vi "Reentrant Display Caller.vi"(9 "card #":dbl, 10 "Stop Button in":bool, 11 "Display Input":T1[](array[typedef])) -> ()   [LabVIEW 2013]
uses:
  Controls/Numeric Indicator.ctl
panel:
  out "VI out":refnum<vi>
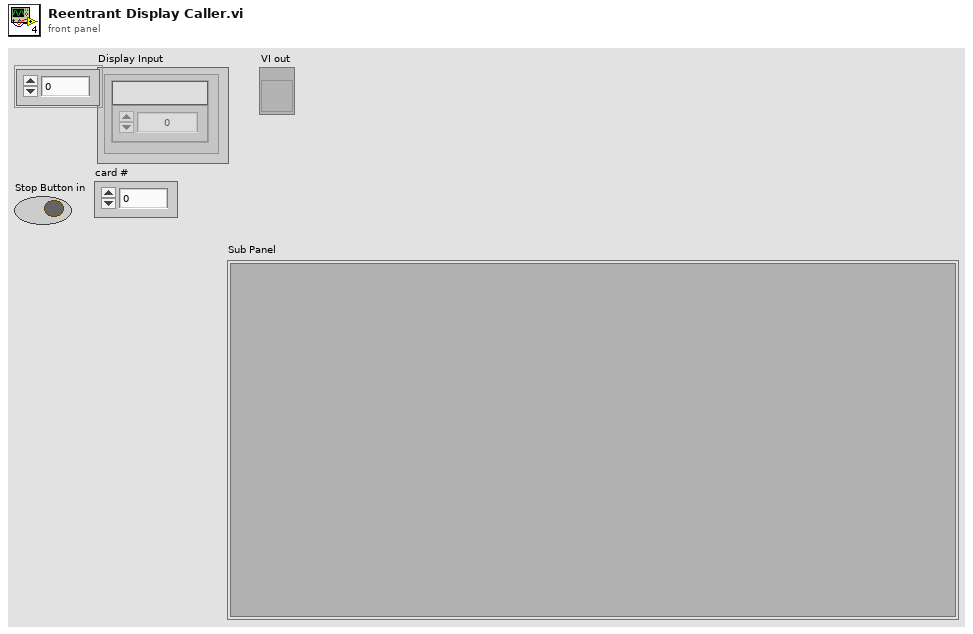
[diagram p1: front panel]
types:
  T1 = typedef "Numeric Indicator.ctl" = cluster{"Numeric Indicator 2":dbl, "String":string}
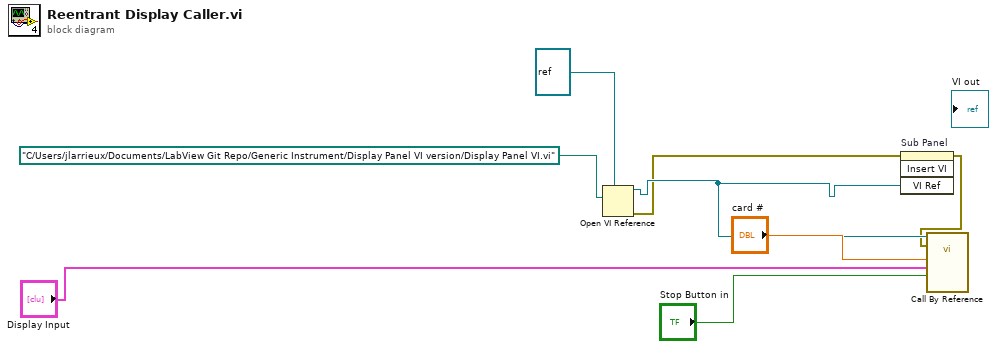
[diagram p0: block diagram]
diagram:
  n1 = Open VI Reference(type specifier VI Refnum (for type only)=refnum<vi> refnum, vi path=path "C:/Users/jlarrieux/Documents/LabView Git Repo/Generic Instrument/Display Panel VI version/Display Panel VI.vi") -> (vi reference=w3:refnum<vi>, error out=w2:errorcluster)  [unwired: 4 in]
  n2 = invoke on="Sub Panel" class="SubPanel" method="Insert VI"(error in=w2, "VI Ref"=w3) -> (error out=w1:errorcluster)  [unwired: 2 in, 3 out]
  n3 = call-by-ref "?"(reference=w3, error in=w1, "Stop Button"="Stop Button in", "Display Input 2"="Display Input", "card #"="card #") -> ()  [unwired: 9 in, 2 out]
